vi "Playback.vi"(8 "error in (no error)":errorcluster, 11 "Replay in":refnum<class "Replay.lvclass">) -> (0 "error out":errorcluster, 3 "Replay out":refnum<class "Replay.lvclass">, 5 "Done?":bool)   [LabVIEW 2016, in "CLD Exam - ATM.lvlib" / "Replay.lvclass"]
uses:
  Replay.lvclass
  Replay.lvclass/Replay.ctl
  Mediator/Classes/Message String/Message String.lvclass
  D:/Repos/Stream/software/Mediator/Classes/Message Interface/Message Interface.lvclass
  Mediator/Classes/Message Transport Queue/Message Transport Queue.lvclass
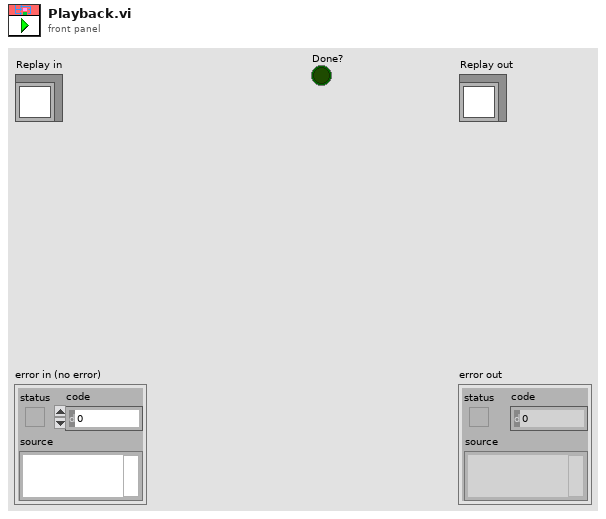
[diagram p1: front panel]
types:
  T1 = cluster{"deltaT":dbl, "Stream":string, "Name":string, "Value":string}[]
  T2 = cluster{"deltaT":dbl, "Stream":string, "Name":string, "Value":string}
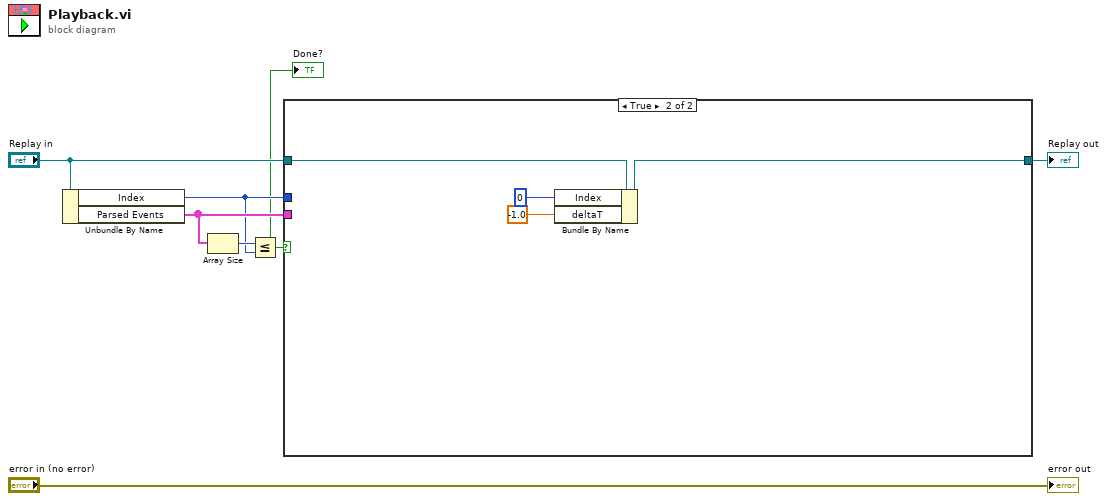
[diagram p0: block diagram]
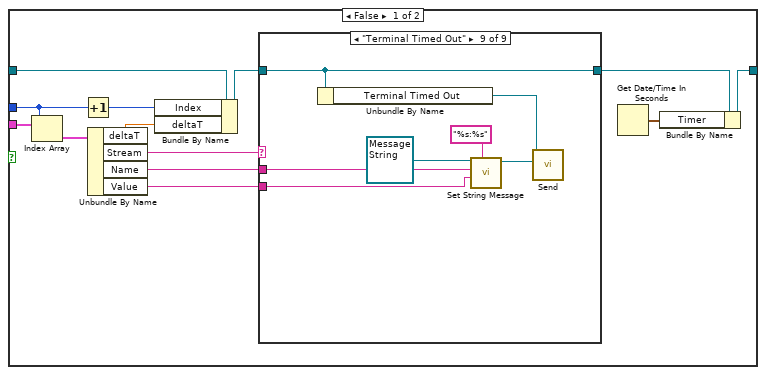
[diagram p2: hidden frame]
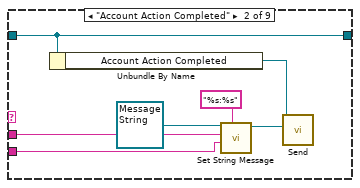
[diagram p4: hidden frame]
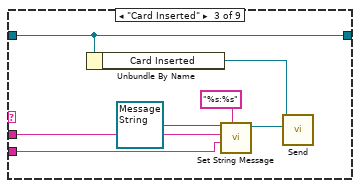
[diagram p5: hidden frame]
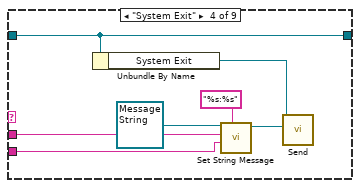
[diagram p6: hidden frame]
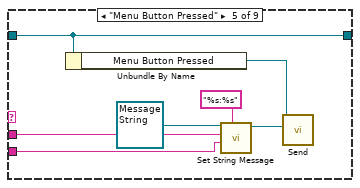
[diagram p7: hidden frame]
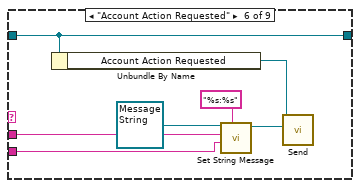
[diagram p8: hidden frame]
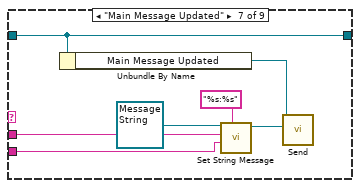
[diagram p9: hidden frame]
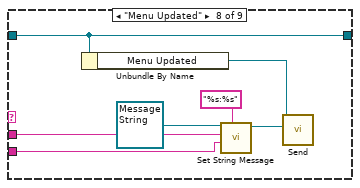
[diagram p10: hidden frame]
diagram:
  n1 = Unbundle By Name("Replay in") -> ("Index"=w4:u32, "Parsed Events"=w6:T1)
  n2 = Array Size(array=w6) -> (size(s)=w5:i32)
  n3 = Less Or Equal?(x=w5, y=w4) -> (x <= y?=w2:bool)
  "Done?" <- w2
  n4 = case shown="True" w2 {
    tunnel: w6 -> [w20 _]
    tunnel: w4 -> [w19 _]
    tunnel: [w10 w78] -> w1
    tunnel: "Replay in" -> [w16 w79]
    frame False {
      n5 = Index Array(array=w20, index=w19) -> (element=w18:T2)
      n6 = Increment(x=w19) -> (x+1=w14:u32)
      n7 = Unbundle By Name(w18) -> ("deltaT"=w13:dbl, "Stream"=w17:string, "Name"=w12:string, "Value"=w11:string)
      n8 = Bundle By Name(cluster=w16, "Index"=w14, "deltaT"=w13) -> (w15:refnum<class "Replay.lvclass">)
      n9 = case shown="\"Terminal Timed Out\"" w17 {
        tunnel: [w21 w25 w32 w39 w46 w53 w60 w67 w74] -> w9
        tunnel: w15 -> [w21 w25 w32 w39 w46 w53 w60 w67 w74]
        tunnel: w12 -> [_ w23 w30 w37 w44 w51 w58 w65 w72]
        tunnel: w11 -> [_ w22 w29 w36 w43 w50 w57 w64 w71]
        frame Default {
        }
        frame "Account Action Completed" {
          n10 = Unbundle By Name(w25) -> ("Account Action Completed"=w24:refnum<class "Message Transport Queue.lvclass">)
          n11 = call "Set String Message.vi"("Format"="%s:%s", "Value"=w22, "Name"=w23, "Message String in"=refnum<class "Message String.lvclass"> refnum) -> ("Message String out"=w27:refnum<class "Message String.lvclass">)  [unwired: 6 in, 1 out]
          n12 = call-dynamic "Send.vi"("Message"=w27, "Message Transport Queue in"=w24) -> ()  [unwired: 7 in, 3 out]
        }
        frame "Card Inserted" {
          n13 = Unbundle By Name(w32) -> ("Card Inserted"=w31:refnum<class "Message Transport Queue.lvclass">)
          n14 = call "Set String Message.vi"("Format"="%s:%s", "Value"=w29, "Name"=w30, "Message String in"=refnum<class "Message String.lvclass"> refnum) -> ("Message String out"=w34:refnum<class "Message String.lvclass">)  [unwired: 6 in, 1 out]
          n15 = call-dynamic "Send.vi"("Message"=w34, "Message Transport Queue in"=w31) -> ()  [unwired: 7 in, 3 out]
        }
        frame "System Exit" {
          n16 = Unbundle By Name(w39) -> ("System Exit"=w38:refnum<class "Message Transport Queue.lvclass">)
          n17 = call "Set String Message.vi"("Format"="%s:%s", "Value"=w36, "Name"=w37, "Message String in"=refnum<class "Message String.lvclass"> refnum) -> ("Message String out"=w41:refnum<class "Message String.lvclass">)  [unwired: 6 in, 1 out]
          n18 = call-dynamic "Send.vi"("Message"=w41, "Message Transport Queue in"=w38) -> ()  [unwired: 7 in, 3 out]
        }
        frame "Menu Button Pressed" {
          n19 = Unbundle By Name(w46) -> ("Menu Button Pressed"=w45:refnum<class "Message Transport Queue.lvclass">)
          n20 = call "Set String Message.vi"("Format"="%s:%s", "Value"=w43, "Name"=w44, "Message String in"=refnum<class "Message String.lvclass"> refnum) -> ("Message String out"=w48:refnum<class "Message String.lvclass">)  [unwired: 6 in, 1 out]
          n21 = call-dynamic "Send.vi"("Message"=w48, "Message Transport Queue in"=w45) -> ()  [unwired: 7 in, 3 out]
        }
        frame "Account Action Requested" {
          n22 = Unbundle By Name(w53) -> ("Account Action Requested"=w52:refnum<class "Message Transport Queue.lvclass">)
          n23 = call "Set String Message.vi"("Format"="%s:%s", "Value"=w50, "Name"=w51, "Message String in"=refnum<class "Message String.lvclass"> refnum) -> ("Message String out"=w55:refnum<class "Message String.lvclass">)  [unwired: 6 in, 1 out]
          n24 = call-dynamic "Send.vi"("Message"=w55, "Message Transport Queue in"=w52) -> ()  [unwired: 7 in, 3 out]
        }
        frame "Main Message Updated" {
          n25 = Unbundle By Name(w60) -> ("Main Message Updated"=w59:refnum<class "Message Transport Queue.lvclass">)
          n26 = call "Set String Message.vi"("Format"="%s:%s", "Value"=w57, "Name"=w58, "Message String in"=refnum<class "Message String.lvclass"> refnum) -> ("Message String out"=w62:refnum<class "Message String.lvclass">)  [unwired: 6 in, 1 out]
          n27 = call-dynamic "Send.vi"("Message"=w62, "Message Transport Queue in"=w59) -> ()  [unwired: 7 in, 3 out]
        }
        frame "Menu Updated" {
          n28 = Unbundle By Name(w67) -> ("Menu Updated"=w66:refnum<class "Message Transport Queue.lvclass">)
          n29 = call "Set String Message.vi"("Format"="%s:%s", "Value"=w64, "Name"=w65, "Message String in"=refnum<class "Message String.lvclass"> refnum) -> ("Message String out"=w69:refnum<class "Message String.lvclass">)  [unwired: 6 in, 1 out]
          n30 = call-dynamic "Send.vi"("Message"=w69, "Message Transport Queue in"=w66) -> ()  [unwired: 7 in, 3 out]
        }
        frame "Terminal Timed Out" {
          n31 = Unbundle By Name(w74) -> ("Terminal Timed Out"=w73:refnum<class "Message Transport Queue.lvclass">)
          n32 = call "Set String Message.vi"("Format"="%s:%s", "Value"=w71, "Name"=w72, "Message String in"=refnum<class "Message String.lvclass"> refnum) -> ("Message String out"=w76:refnum<class "Message String.lvclass">)  [unwired: 6 in, 1 out]
          n33 = call-dynamic "Send.vi"("Message"=w76, "Message Transport Queue in"=w73) -> ()  [unwired: 7 in, 3 out]
        }
      }
      n34 = Get Date/Time In Seconds() -> (seconds since 1Jan1904=w8:timestamp)
      n35 = Bundle By Name(cluster=w9, "Timer"=w8) -> (w10:refnum<class "Replay.lvclass">)
    }
    frame True {
      n36 = Bundle By Name(cluster=w79, "Index"=u32 0, "deltaT"=-1.0) -> (w78:refnum<class "Replay.lvclass">)
    }
  }
  "Replay out" <- w1
  "error out" <- "error in (no error)"
